vi "LAUNCHBALL2.vi"   [LabVIEW 2016, in "Test2.lvrbt"]
uses:
  Test2.lvrbt
  <vilib>/NXT/Hardware/Plugins/Tetrix DC Motor/TetrixDCMotorAddress.ctl
  <vilib>/NXT/Hardware/Plugins/Tetrix 180 deg Servo/Tetrix180ServoAddress.ctl
  <vilib>/NXT/NXTIO Xnodes/NXTIONodeSubVIs/TETRIX IO Move Servos.vi
  <vilib>/NXT/Dual Mode Library/Waits/Wait_Num.vi
  <vilib>/NXT/NXTIO Xnodes/NXTIONodeSubVIs/TETRIX IO Move DC Motors.vi
  <vilib>/NXT/NXTIO Xnodes/NXTIONodeSubVIs/TETRIX IO Stop DC Motors.vi
  <vilib>/NXT/NXTIO Xnodes/AddressXNode/NXTIOAddress.xnode
  <vilib>/NXT/Subs/LVHSConnector.ctl
  <vilib>/NXT/NXTIO Xnodes/NXTIOXNode/NXTIO.xnode
  <vilib>/NXT/LegoClasses/BrickReference/BrickReference.lvclass
types:
  T1 = typedef "Tetrix180ServoAddress.ctl" = i32
  T2 = cluster{"Tetrix180Servo":T1, "Tetrix180Servo":T1, "Tetrix180Servo":T1, "Tetrix180Servo":T1, "Tetrix180Servo":T1, "Tetrix180Servo":T1}
  T3 = typedef "LVHSConnector.ctl" = refnum<class "BrickReference.lvclass">
  T4 = typedef "TetrixDCMotorAddress.ctl" = i32
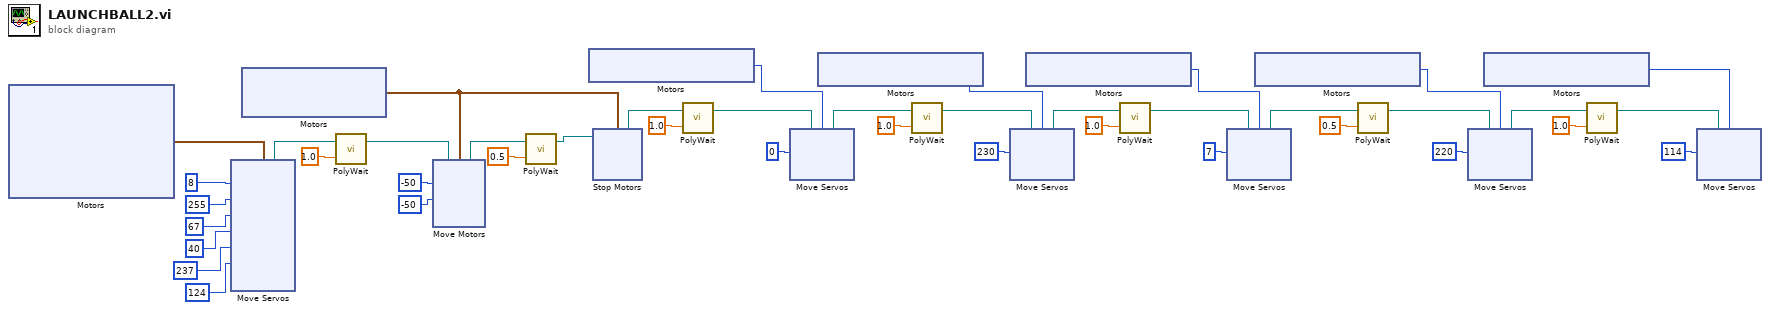
[diagram p0: block diagram]
diagram:
  n1 = xnode "Motors"() -> ("Motor"=w35:T2)
  n2 = xnode "Move Servos"("Position 6"=u8 124, "Position 5"=u8 237, "Position 4"=u8 40, "Position 3"=u8 67, "Position 2"=u8 255, "Position 1"=u8 8, "Motors"=w35) -> ("NXT/EV3"=w27:T3)  [unwired: 1 in]
  n3 = xnode "Motors"() -> ("Motor"=w36:cluster{"TetrixDCMotor":T4, "TetrixDCMotor":T4})
  n4 = call-poly <vilib>:"PolyWait.vi"("Time (1 sec)"=sgl 1.0, "NXT/EV3"=w27) -> ("NXT/EV3"=w26:T3)  [unwired: 2 in]
  n5 = xnode "Move Motors"("Power/Speed 2"=i8 -50, "Power/Speed 1"=i8 -50, "Motors"=w36, "NXT/EV3"=w26) -> ("NXT/EV3"=w39:T3)
  n6 = call-poly <vilib>:"PolyWait.vi"("Time (1 sec)"=sgl 0.5, "NXT/EV3"=w39) -> ("NXT/EV3"=w37:T3)  [unwired: 2 in]
  n7 = xnode "Motors"() -> ("Motor"=w22:T1)
  n8 = xnode "Stop Motors"("Motors"=w36, "NXT/EV3"=w37) -> ("NXT/EV3"=w25:T3)
  n9 = call-poly <vilib>:"PolyWait.vi"("Time (1 sec)"=sgl 1.0, "NXT/EV3"=w25) -> ("NXT/EV3"=w23:T3)  [unwired: 2 in]
  n10 = xnode "Move Servos"("Position 1"=u8 0, "Motors"=w22, "NXT/EV3"=w23) -> ("NXT/EV3"=w16:T3)
  n11 = xnode "Motors"() -> ("Motor"=w18:T1)
  n12 = call-poly <vilib>:"PolyWait.vi"("Time (1 sec)"=sgl 1.0, "NXT/EV3"=w16) -> ("NXT/EV3"=w19:T3)  [unwired: 2 in]
  n13 = xnode "Move Servos"("Position 1"=u8 230, "Motors"=w18, "NXT/EV3"=w19) -> ("NXT/EV3"=w11:T3)
  n14 = xnode "Motors"() -> ("Motor"=w13:T1)
  n15 = call-poly <vilib>:"PolyWait.vi"("Time (1 sec)"=sgl 1.0, "NXT/EV3"=w11) -> ("NXT/EV3"=w14:T3)  [unwired: 2 in]
  n16 = xnode "Move Servos"("Position 1"=u8 7, "Motors"=w13, "NXT/EV3"=w14) -> ("NXT/EV3"=w6:T3)
  n17 = xnode "Motors"() -> ("Motor"=w8:T1)
  n18 = call-poly <vilib>:"PolyWait.vi"("Time (1 sec)"=sgl 0.5, "NXT/EV3"=w6) -> ("NXT/EV3"=w9:T3)  [unwired: 2 in]
  n19 = xnode "Move Servos"("Position 1"=u8 220, "Motors"=w8, "NXT/EV3"=w9) -> ("NXT/EV3"=w1:T3)
  n20 = xnode "Motors"() -> ("Motor"=w3:T1)
  n21 = call-poly <vilib>:"PolyWait.vi"("Time (1 sec)"=sgl 1.0, "NXT/EV3"=w1) -> ("NXT/EV3"=w4:T3)  [unwired: 2 in]
  n22 = xnode "Move Servos"("Position 1"=u8 114, "Motors"=w3, "NXT/EV3"=w4) -> ()  [unwired: 1 out]
